vi "AppConfigXMLToType.vi"(8 "error in (no error)":errorcluster, 10 "Config in":variant, 11 "ModelValidation in":refnum<class "ModelValidationPlugin.lvclass">) -> (0 "error out":errorcluster, 3 "ModelValidation out":refnum<class "ModelValidationPlugin.lvclass">)   [LabVIEW 2014, in "AppPlugins.lvlib" / "ModelValidationPlugin.lvclass"]
uses:
  ModelValidationPlugin.lvclass
  PublicAPI/TypeDef/Config.ctl
  ModelValidationPlugin.lvclass/ModelValidationPlugin.ctl
  Accessors/Write ModelValidationConfig.vi
  <vilib>/Utility/error.llb/Error Cluster From Error Code.vi
  <vilib>/ErrorRing/Error Ring.xnode
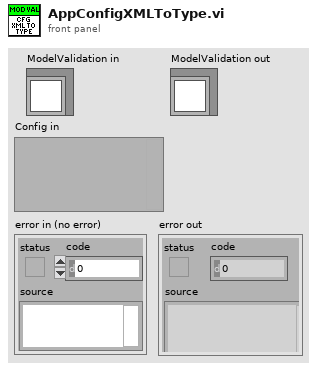
[diagram p1: front panel]
types:
  T1 = typedef "AppPlugins.lvlib/ModelValidationPlugin.lvclass/Config.ctl" = cluster{"NoiseVariance":dbl, "Iindex":i32, "OffsetTime":dbl, "InterpolationFactor":i32, "Initial condition":cluster{"H0":dbl, "xd0":dbl, "D0":dbl}}
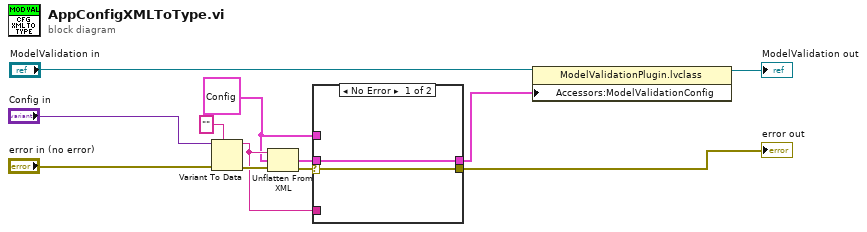
[diagram p0: block diagram]
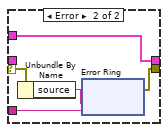
[diagram p2: hidden frame]
diagram:
  w1 = T1 {"NoiseVariance"=0.001, "Iindex"=3, "OffsetTime"=2.0, "InterpolationFactor"=4, "Initial condition"={"H0"=4.55, "xd0"=0.275, "D0"=4.2}} ("ModelValidationConfig")
  n1 = Variant To Data(error in="error in (no error)", type="", Variant="Config in") -> (data=w8:string, error out=w11:errorcluster)
  n2 = Unflatten From XML(xml string=w8, type=w1, error in (no error)=w11) -> (value=w9:T1, error out=w10:errorcluster)
  n3 = case shown="No Error" w10 {
    selector: w10 -> [w13 w18]
    tunnel: w9 -> [w14 _]
    tunnel: [w14 w19] -> w2
    tunnel: [w13 w15] -> w5
    tunnel: w1 -> [_ w19]
    tunnel: w8 -> [_ w16]
    frame No Error {
    }
    frame Error {
      n4 = Unbundle By Name(w18) -> ("source"=w17:string)
      n5 = xnode "Error Ring"("parameter 0"=w17, "parameter 1"=w16) -> ("error out"=w15:errorcluster)
    }
  }
  "error out" <- w5
  n6 = property class="ModelValidationPlugin.lvclass"(reference="ModelValidation in", "Accessors:ModelValidationConfig"=w2) -> (reference out=→"ModelValidation out":refnum<class "ModelValidationPlugin.lvclass">)  [unwired: 1 in, 1 out]
